vi "Main.vi"(8 "error in (no error)":errorcluster, 11 "Cascade512Base in":refnum<class "DAQCascade512.lvclass">) -> (0 "error out":errorcluster, 3 "component":refnum<class "DAQCascade512.lvclass">)   [LabVIEW 2012, in "DAQCascade512.lvclass"]
doc: "Main VI of the component."
uses:
  DAQCascade512.lvclass
  <vilib>/Distrio/Murmex/Murmex/command_enum.ctl
  <vilib>/Distrio/Murmex/InitialiseMessage/InitialiseMessage class.ctl
  <vilib>/Distrio/Murmex/InitialiseMessage/InitialiseMessage.lvclass
  DAQCascade512.lvclass/DAQCascade512.ctl
  <vilib>/Distrio/Murmex/TerminateMessage/TerminateMessage class.ctl
  <vilib>/Distrio/Murmex/TerminateMessage/TerminateMessage.lvclass
  <vilib>/Distrio/Murmex/ConfigureMessage/ConfigureMessage.lvclass
  <vilib>/Distrio/Murmex/StartMessage/StartMessage.lvclass
  <vilib>/Distrio/Murmex/StopMessage/StopMessage.lvclass
  <vilib>/Distrio/Murmex/Murmex/Set configure at initialise.vi
  <vilib>/Distrio/Murmex/Murmex/Set log reference.vi
  <vilib>/Distrio/Murmex/Murmex/Set VI reference.vi
  <vilib>/Distrio/Murmex/Murmex/Murmex.lvclass
  <vilib>/Distrio/Murmex/Message/Message.lvclass
panel:
  in  "image handles":u32[](array[numeric])
  in  "button:acquire":bool
  in  "button:stop":bool
  in  "button:start":bool
  out "img":sgl[][](graph)
  in  "button:configure":bool
  in  "Tab Control":enum32{"Settings", "Debug", "About"}(tab)
  in  "exposure":dbl=0.01 format="%.3f"
  in  "number of images":u32=1000
  out "Log":string
  out "generic command":string
  in  "command":T1
  in  "component ID":string
  in  "button:send":bool
  in  "quit":bool
  out "terminate?":bool
  # "camera made by Ali"
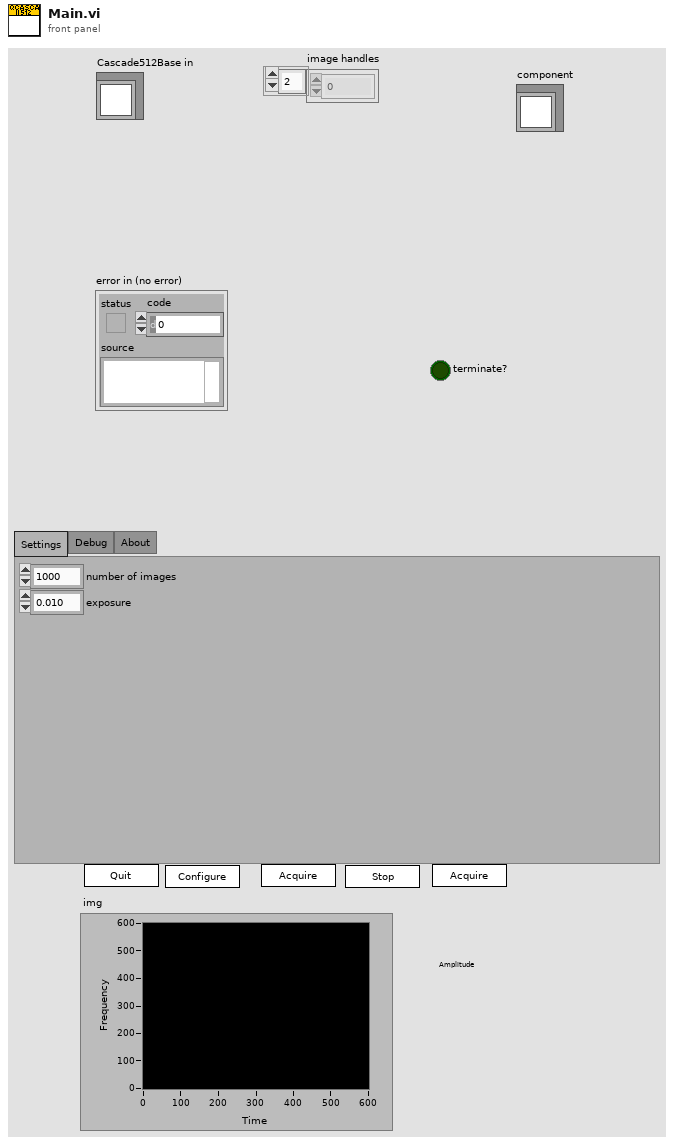
[diagram p1: front panel]
types:
  T1 = typedef "Murmex.lvlib/Murmex.lvclass/command_enum.ctl" = enum16{"null", "initialise", "reset", "terminate", "acknowledge", "update", "inspect", "inform", "proceed", "start", "stop", "fetch", "configure", "generic"}
  T2 = typedef "Murmex.lvlib/InitialiseMessage.lvclass/InitialiseMessage class.ctl" = refnum<class "InitialiseMessage.lvclass">
  T3 = typedef "Murmex.lvlib/TerminateMessage.lvclass/TerminateMessage class.ctl" = refnum<class "TerminateMessage.lvclass">
  T4 = typedef "Image_type.ctl" = u32
  T5 = typedef "Murmex.lvlib/Murmex.lvclass/Event type enumerations.ctl" = enum16{"before", "after"}
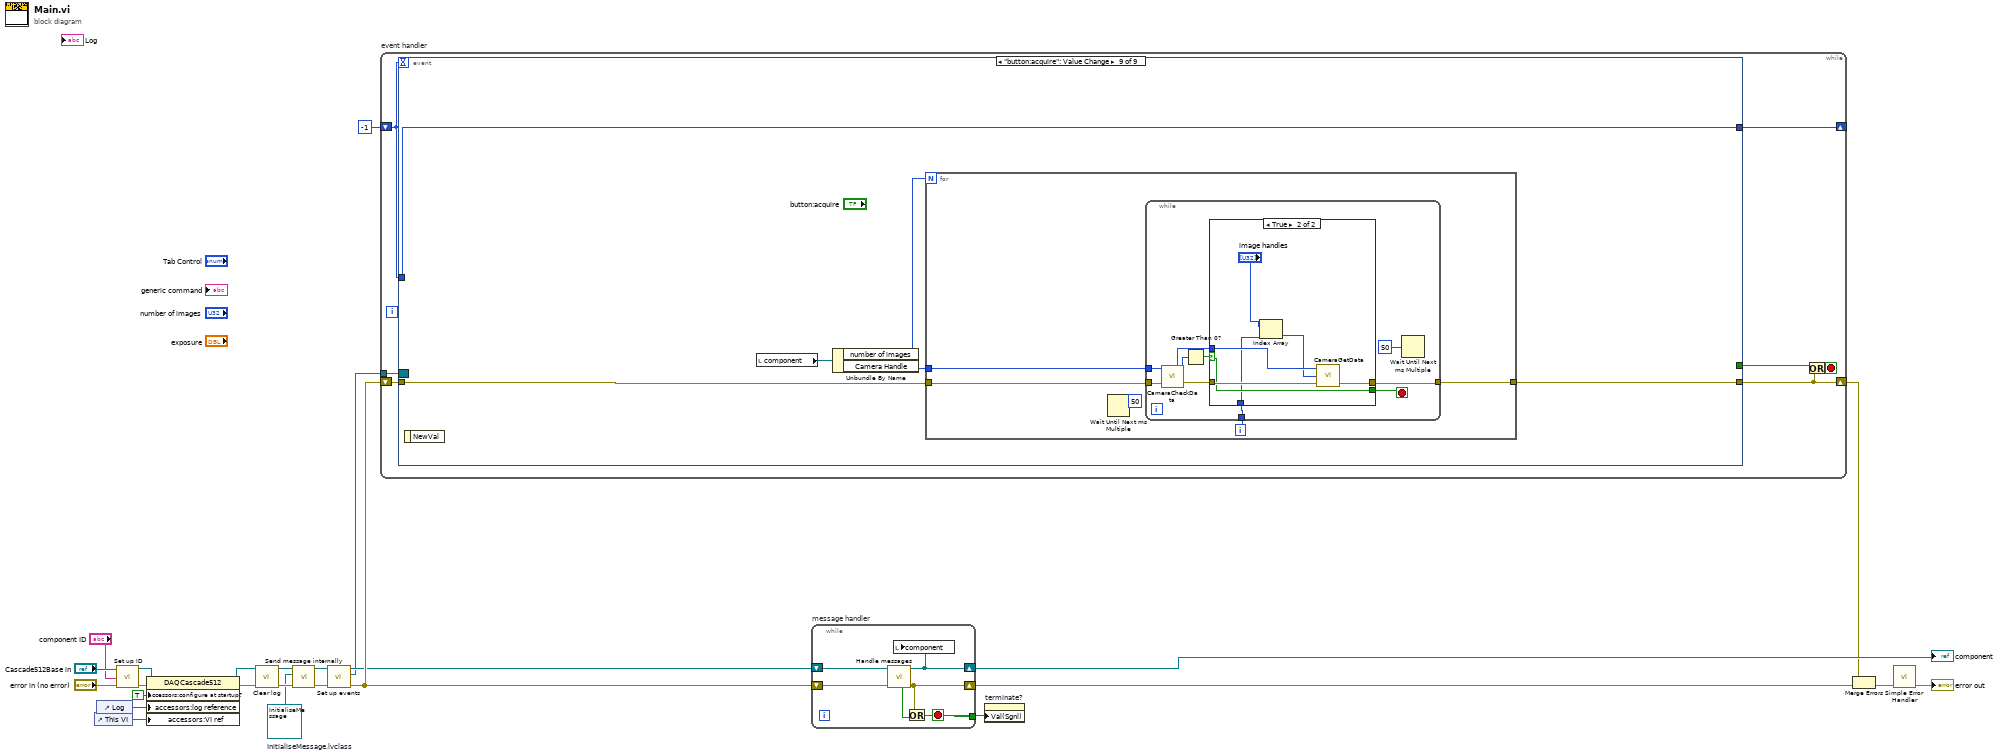
[diagram p0: block diagram]
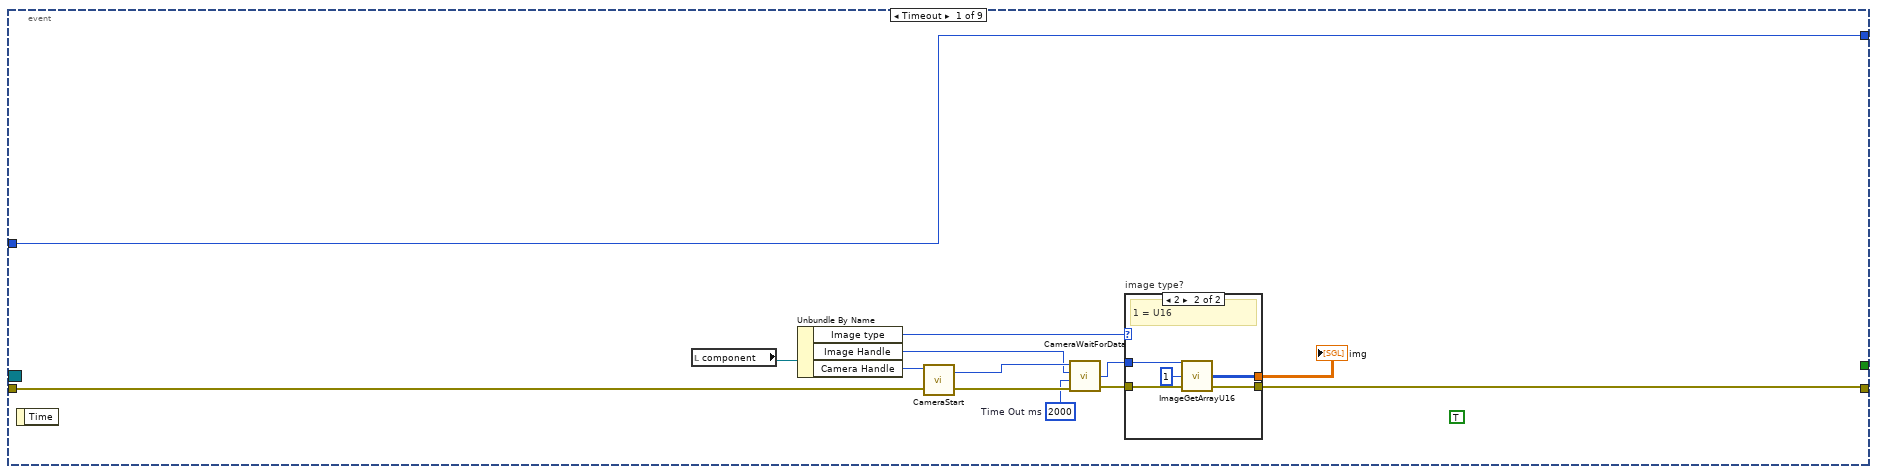
[diagram p2: hidden frame]
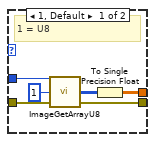
[diagram p3: hidden frame]
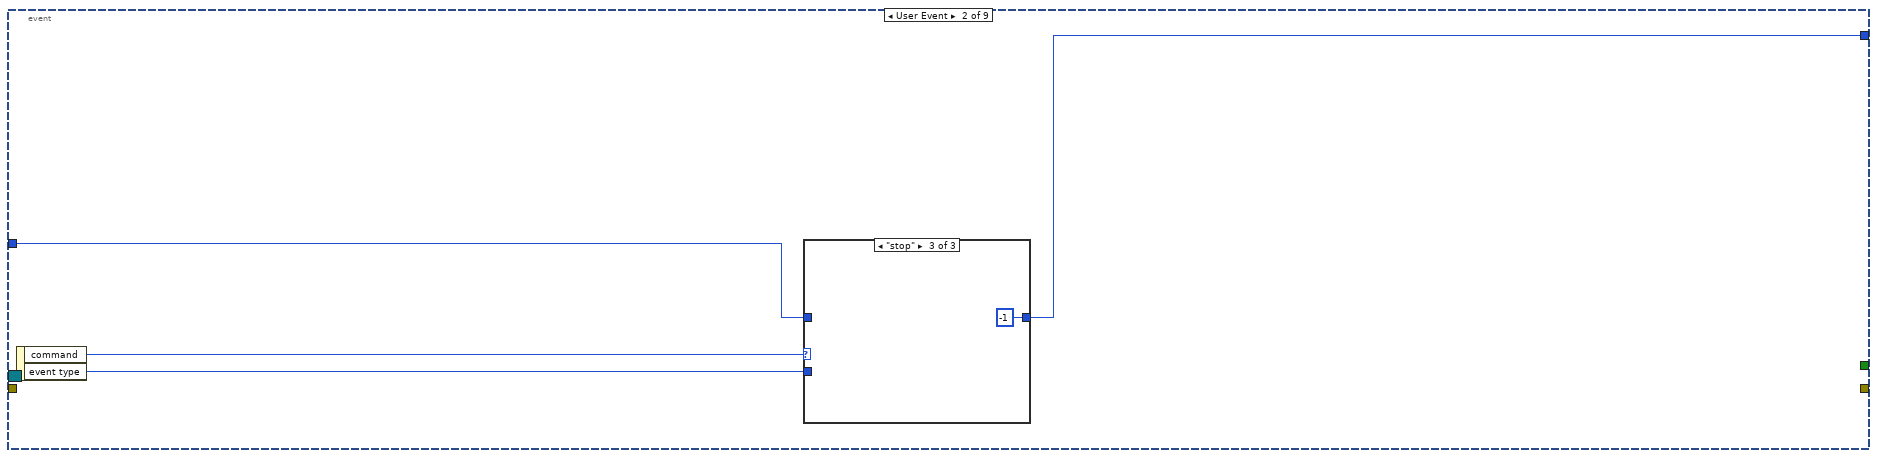
[diagram p4: hidden frame]
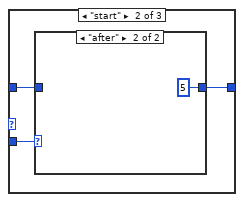
[diagram p6: hidden frame]
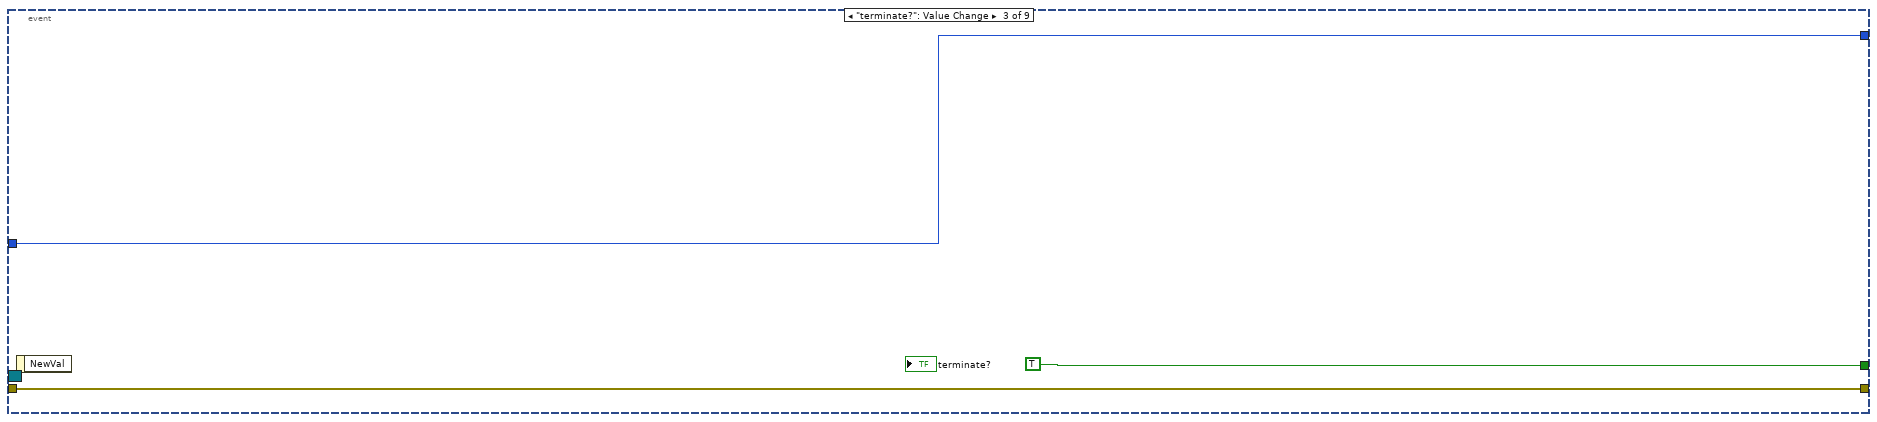
[diagram p8: hidden frame]
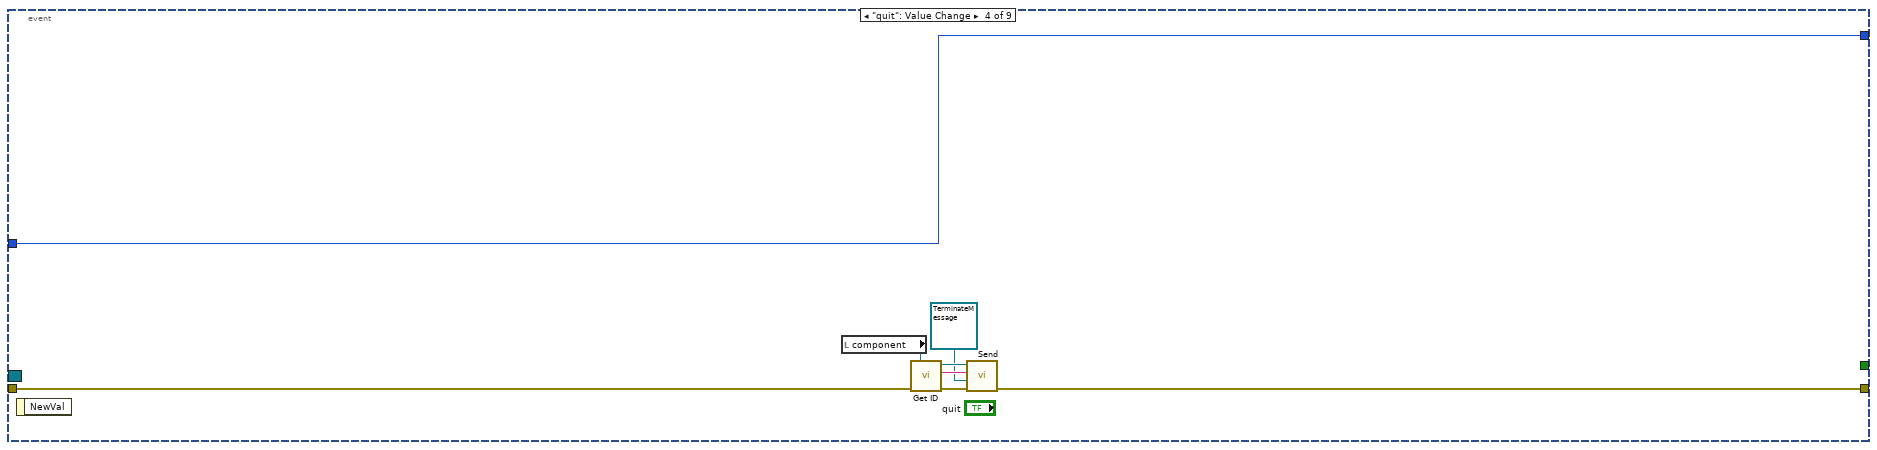
[diagram p9: hidden frame]
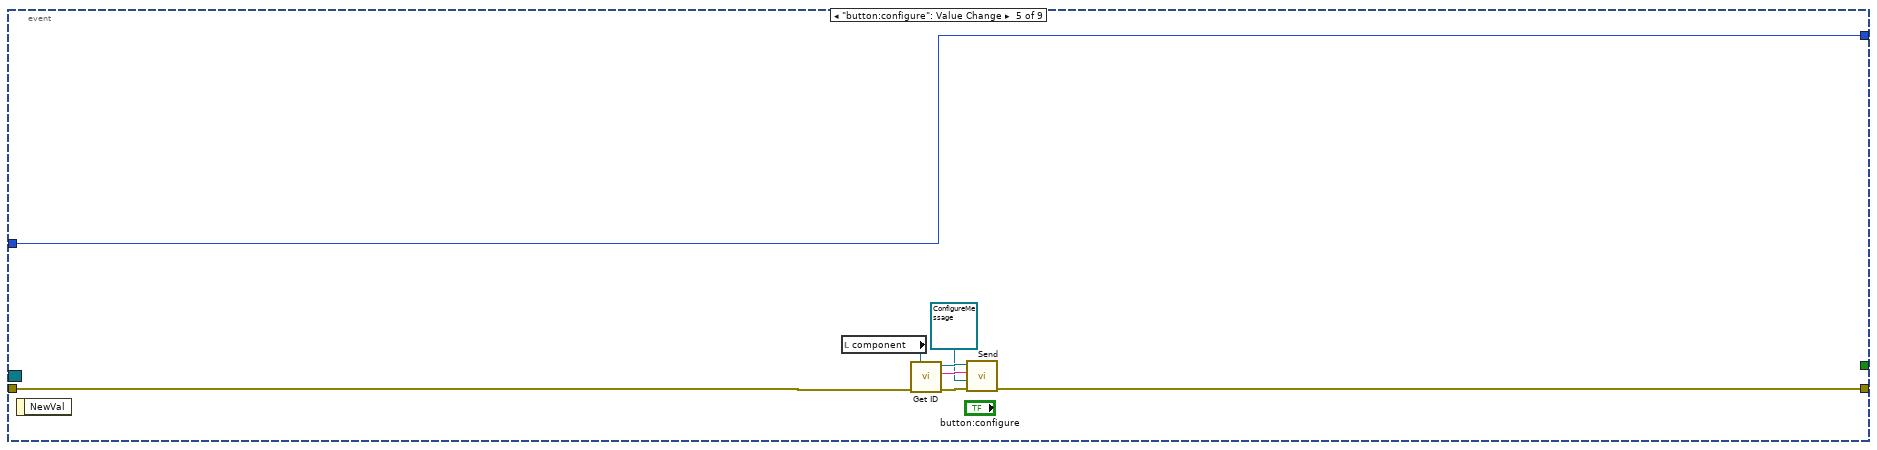
[diagram p10: hidden frame]
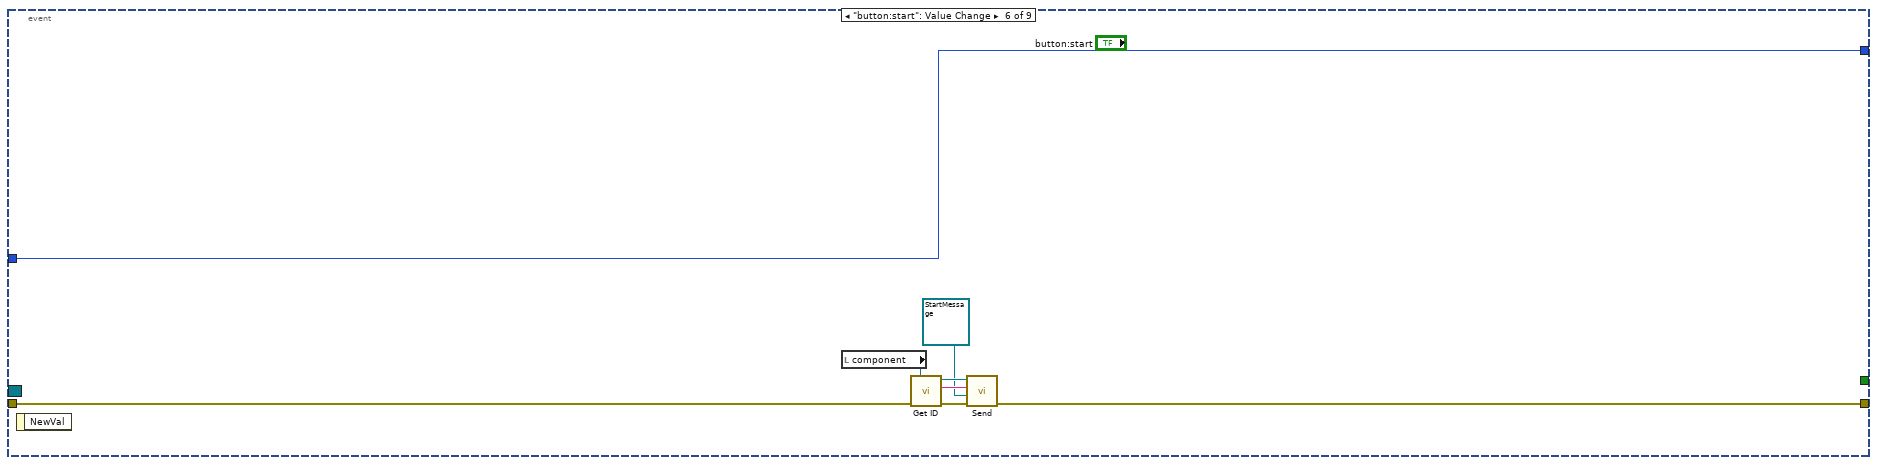
[diagram p11: hidden frame]
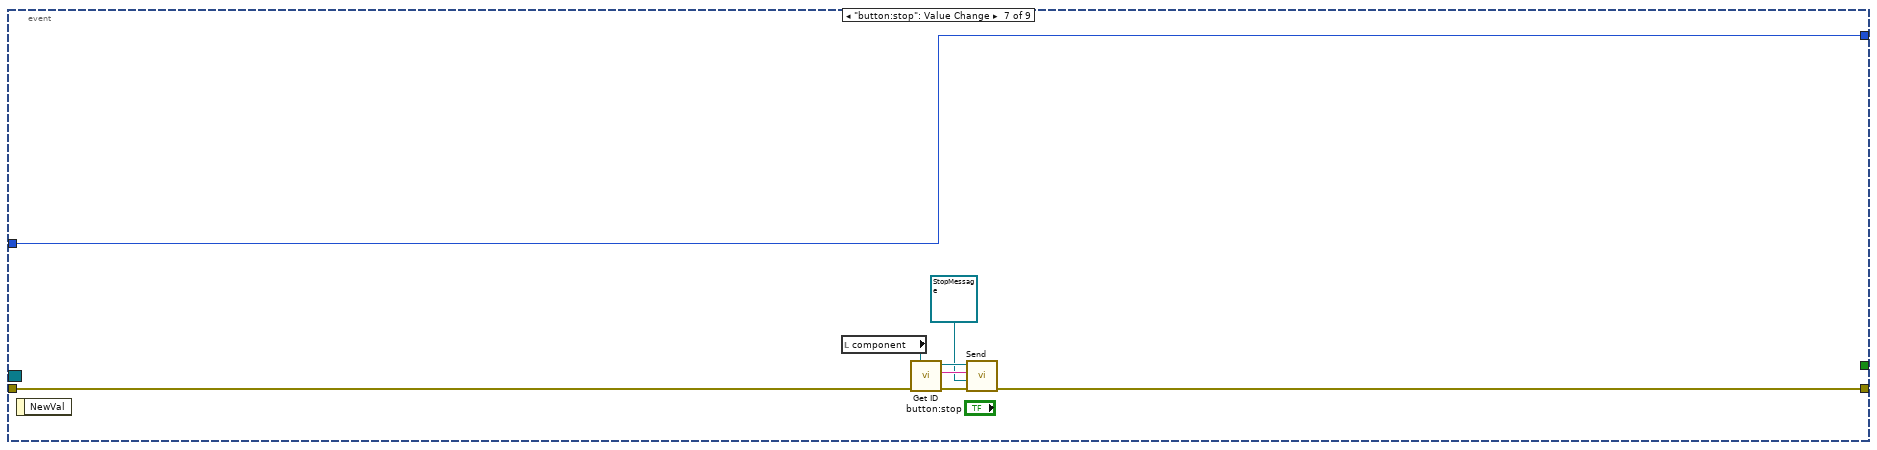
[diagram p12: hidden frame]
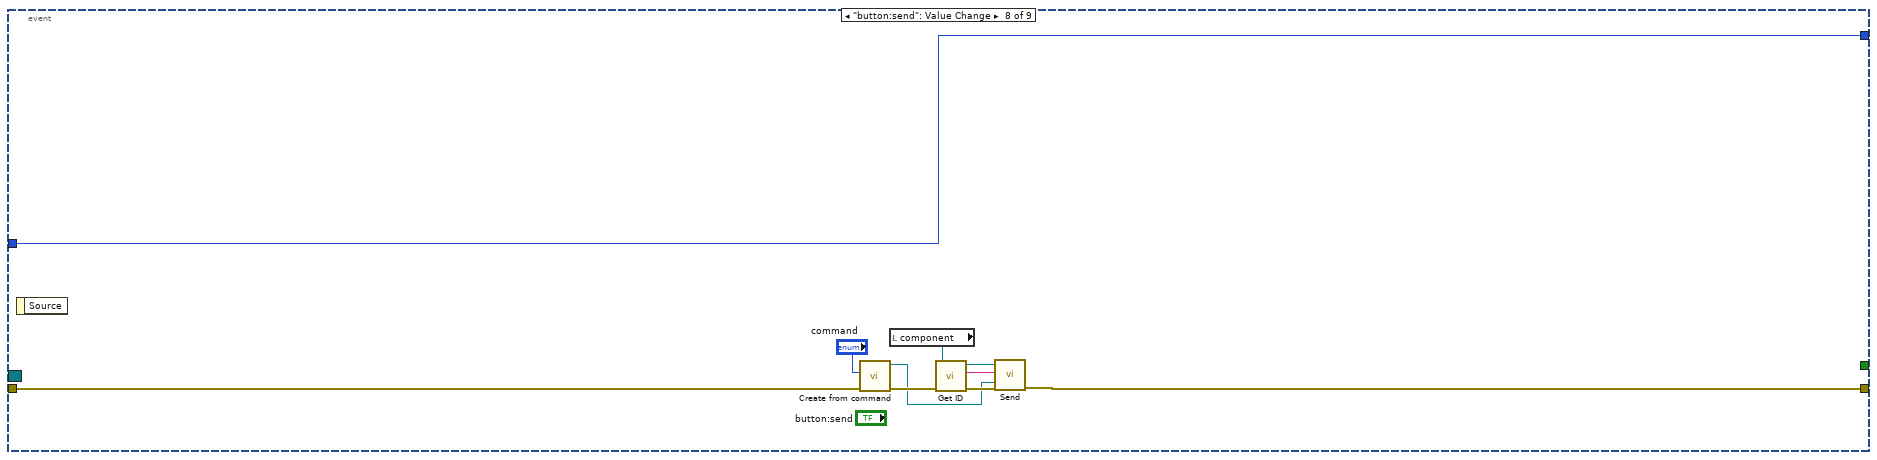
[diagram p13: hidden frame]
diagram:
  w17 = T2 refnum  # InitialiseMessage.lvclass
  n1 = control-ref of="This VI"() -> (w23:refnum<vi>)
  n2 = control-ref of="Log"() -> (w22:refnum<vi>)
  n3 = call <vilib>:"Set up ID.vi"("error in (no error)"="error in (no error)", "component ID"="component ID", "MurmexBase in"="Cascade512Base in") -> ("error out"=w13:errorcluster, "MurmexBase out"=w15:refnum<class "DAQCascade512.lvclass">)  [unwired: 6 in, 1 out]
  n4 = property class="DAQCascade512"(reference=w15, error in=w13, "accessors:configure at startup?"=TRUE, "accessors:log reference"=w22, "accessors:VI ref"=w23) -> (reference out=w21:refnum<class "DAQCascade512.lvclass">, error out=w20:errorcluster)
  n5 = call <vilib>:"Clear log.vi"("error in (no error)"=w20, "MurmexBase in"=w21) -> ("error out"=w18:errorcluster, "MurmexBase out"=w19:refnum<class "DAQCascade512.lvclass">)  [unwired: 8 in]
  n6 = call <vilib>:"Send message internally.vi"("error in (no error)"=w18, "Message"=w17, "Murmex in"=w19) -> ("error out"=w6:errorcluster, "Murmex out"=w4:refnum<class "DAQCascade512.lvclass">)  [unwired: 7 in]
  n7 = call <vilib>:"Set up events.vi"("error in (no error)"=w6, "MurmexBase in"=w4) -> ("error out"=w5:errorcluster, "Event Registration Refnum"=w2:refnum<event-registration>, "MurmexBase out"=w3:refnum<class "DAQCascade512.lvclass">)  [unwired: 7 in]
  n8 = while "event handler" {
    shift-right: [w29] -> w10
    shift-left: w5 -> [w31]
    tunnel: w2 -> [w28]
    shift-right: [w26] -> _
    shift-left: -1 -> [w27]
    stop <- w32 stop-if-true
    n9 = event shown="[8] \"button:acquire\": Value Change" {
      selector: w28 -> [_ _ _ _ _ _ _ _ _]
      dyn-events: _ -> [_ _ _ _ _ _ _ _ _]
      timeout: w27 -> [_ _ _ _ _ _ _ _ _]
      tunnel: [_ _ TRUE _ _ _ _ _ _] -> w30
      tunnel: w31 -> [w43 _ w69 w76 w84 w92 w100 w111 w117]
      tunnel: [w42 _ w69 w75 w83 w91 w99 w108 w116] -> w29
      tunnel: w27 -> [w45 w58 w68 w71 w79 w88 w96 w103 w118]
      tunnel: [w45 w57 w68 w71 w79 w88 w96 w103 w118] -> w26
      event Timeout {
        w36 = u32 2000  # Time Out ms
        (unwired) TRUE
        n10 = event-data() -> ()  [unwired: 1 in, 1 out]
        n11 = local read "component"() -> (w44:refnum<class "DAQCascade512.lvclass">)
        n12 = Unbundle By Name(w44) -> ("Image type"=w37:T4, "Image Handle"=w38:u32, "Camera Handle"=w40:u32)
        n13 = call <userlib>:"CameraStart.vi"("error in"=w43, "Camera Handle"=w40) -> ("error out"=w41:errorcluster, "Camera Handle"=w39:u32)
        n14 = call <userlib>:"CameraWaitForData.vi"("error in"=w41, "Time Out ms"=w36, "Image Handle"=w38, "Camera Handle"=w39) -> ("error out"=w35:errorcluster, "Image Handle"=w34:u32)  [unwired: 1 out]
        n15 = case "image type?" shown="2" w37 {
          tunnel: [w51 w56] -> w42
          tunnel: [w47 w55] -> w33
          tunnel: w35 -> [w49 w54]
          tunnel: w34 -> [w48 w53]
          frame 1, Default {
            # "1 = U8"
            n16 = call <userlib>:"ImageGetArrayU8.vi"("error in (no error)"=w49, "Z Position"=u32 1, "Image Handle"=w48) -> ("error out"=w51:errorcluster, "Array"=w50:u8[][])  [unwired: 1 out]
            n17 = To Single Precision Float(number=w50) -> (single precision float=w47:sgl[][])
          }
          frame 2 {
            # "1 = U16"
            n18 = call <userlib>:"ImageGetArrayU16.vi"("error in"=w54, "Z position"=u32 1, "Image Handle"=w53) -> ("error out"=w56:errorcluster, "Array uint 16"=w55:u16[][])  [unwired: 1 out]
          }
        }
        "img" <- w33
      }
      event User Event {
        n19 = event-data() -> ("command"=w60:T1, "event type"=w59:T5)  [unwired: 1 in]
        n20 = case shown="\"stop\"" w60 {
          tunnel: w59 -> [_ w64 _]
          tunnel: w58 -> [w61 w63 _]
          tunnel: [w61 w62 -1] -> w57
          frame Default {
          }
          frame "start" {
            n21 = case shown="\"after\"" w64 {
              tunnel: w63 -> [w65 _]
              tunnel: [w65 5] -> w62
              frame "before", Default {
              }
              frame "after" {
              }
            }
          }
          frame "stop" {
          }
        }
      }
      event "terminate?": Value Change {
        n22 = event-data() -> ()  [unwired: 1 in, 1 out]
      }
      event "quit": Value Change {
        n23 = event-data() -> ()  [unwired: 1 in, 1 out]
        n24 = local read "component"() -> (w74:refnum<class "DAQCascade512.lvclass">)
        n25 = call <vilib>:"Get ID.vi"("error in (no error)"=w76, "Murmex in"=w74) -> ("error out"=w78:errorcluster, "component id"=w73:string, "Murmex out"=w77:refnum<class "DAQCascade512.lvclass">)  [unwired: 7 in]
        n26 = call <vilib>:"Send.vi"("error in (no error)"=w78, "Message"=T3 refnum ("TerminateMessage.lvclass"), "recipient"=w73, "Murmex in"=w77) -> ("error out"=w75:errorcluster)  [unwired: 6 in, 1 out]
      }
      event "button:configure": Value Change {
        n27 = event-data() -> ()  [unwired: 1 in, 1 out]
        n28 = local read "component"() -> (w82:refnum<class "DAQCascade512.lvclass">)
        n29 = call <vilib>:"Get ID.vi"("error in (no error)"=w84, "Murmex in"=w82) -> ("error out"=w86:errorcluster, "component id"=w81:string, "Murmex out"=w85:refnum<class "DAQCascade512.lvclass">)  [unwired: 7 in]
        n30 = call <vilib>:"Send.vi"("error in (no error)"=w86, "Message"=refnum<class "ConfigureMessage.lvclass"> refnum ("Distrio Murmex 1.5:ConfigureMessage"), "recipient"=w81, "Murmex in"=w85) -> ("error out"=w83:errorcluster)  [unwired: 6 in, 1 out]
      }
      event "button:start": Value Change {
        n31 = event-data() -> ()  [unwired: 1 in, 1 out]
        n32 = local read "component"() -> (w90:refnum<class "DAQCascade512.lvclass">)
        n33 = call <vilib>:"Get ID.vi"("error in (no error)"=w92, "Murmex in"=w90) -> ("error out"=w94:errorcluster, "component id"=w89:string, "Murmex out"=w93:refnum<class "DAQCascade512.lvclass">)  [unwired: 7 in]
        n34 = call <vilib>:"Send.vi"("error in (no error)"=w94, "Message"=refnum<class "StartMessage.lvclass"> refnum ("Distrio Murmex 1.5:StartMessage"), "recipient"=w89, "Murmex in"=w93) -> ("error out"=w91:errorcluster)  [unwired: 6 in, 1 out]
      }
      event "button:stop": Value Change {
        n35 = event-data() -> ()  [unwired: 1 in, 1 out]
        n36 = local read "component"() -> (w98:refnum<class "DAQCascade512.lvclass">)
        n37 = call <vilib>:"Get ID.vi"("error in (no error)"=w100, "Murmex in"=w98) -> ("error out"=w102:errorcluster, "component id"=w97:string, "Murmex out"=w101:refnum<class "DAQCascade512.lvclass">)  [unwired: 7 in]
        n38 = call <vilib>:"Send.vi"("error in (no error)"=w102, "Message"=refnum<class "StopMessage.lvclass"> refnum ("Distrio Murmex 1.5:StopMessage"), "recipient"=w97, "Murmex in"=w101) -> ("error out"=w99:errorcluster)  [unwired: 6 in, 1 out]
      }
      event "button:send": Value Change {
        n39 = event-data() -> ()  [unwired: 1 in, 1 out]
        n40 = call <vilib>:"Create from command.vi"("error in (no error)"=w111, "command"="command") -> ("error out"=w110:errorcluster, "Message out"=w106:refnum<class "Message.lvclass">)  [unwired: 8 in]
        n41 = local read "component"() -> (w107:refnum<class "DAQCascade512.lvclass">)
        n42 = call <vilib>:"Get ID.vi"("error in (no error)"=w110, "Murmex in"=w107) -> ("error out"=w109:errorcluster, "component id"=w104:string, "Murmex out"=w105:refnum<class "DAQCascade512.lvclass">)  [unwired: 7 in]
        n43 = call <vilib>:"Send.vi"("error in (no error)"=w109, "Message"=w106, "recipient"=w104, "Murmex in"=w105) -> ("error out"=w108:errorcluster)  [unwired: 6 in, 1 out]
      }
      event "button:acquire": Value Change {
        n44 = event-data() -> ()  [unwired: 1 in, 1 out]
        n45 = local read "component"() -> (w115:refnum<class "DAQCascade512.lvclass">)
        n46 = Unbundle By Name(w115) -> ("number of images"=w114:u32, "Camera Handle"=w113:u32)
        n47 = for {
          N: w114 -> [_]
          tunnel: w117 -> [w123]
          tunnel: [w120] -> w116
          tunnel: w113 -> [w119]
          i -> [w121]
          n48 = Wait Until Next ms Multiple(millisecond multiple=u32 50) -> ()  [unwired: 1 out]
          n49 = while {
            tunnel: w123 -> [w132]
            tunnel: w119 -> [w131]
            tunnel: [w126] -> w120
            tunnel: w121 -> [w124]
            stop <- w127 stop-if-true
            n50 = call <userlib>:"CameraCheckData.vi"("Camera Handle"=w131, "error in"=w132) -> ("Camera Handle"=w129:u32, "Number Of Frames Available"=w133:i32, "error out"=w128:errorcluster)
            n51 = Greater Than 0?(x=w133) -> (x > 0?=w130:bool)
            n52 = case shown="True" w130 {
              selector: w130 -> [w134 w140]
              tunnel: w129 -> [_ w142]
              tunnel: w128 -> [w135 w141]
              tunnel: [w134 w140] -> w127
              tunnel: [w135 w139] -> w126
              tunnel: w124 -> [_ w138]
              frame False {
              }
              frame True {
                n53 = Index Array(array="image handles", index=w138) -> (element=w136:u32)
                n54 = call <userlib>:"CameraGetData.vi"("error in"=w141, "Data Handle"=w136, "Camera Handle"=w142) -> ("error out"=w139:errorcluster)  [unwired: 2 out]
              }
            }
            n55 = Wait Until Next ms Multiple(millisecond multiple=u32 50) -> ()  [unwired: 1 out]
          }
        }
      }
    }
    n56 = Or(x=w30, y=w29) -> (x .or. y?=w32:bool)
  }
  n57 = while "message handler" {
    shift-right: [w143] -> w25
    shift-left: w3 -> [w147]
    shift-right: [w146] -> w9
    shift-left: w5 -> [w148]
    tunnel: [w144] -> w12
    stop <- w144 stop-if-true
    n58 = call <vilib>:"Handle messages.vi"("error in (no error)"=w148, "Murmex in"=w147) -> ("error out"=w146:errorcluster, "Murmex out"=w143:refnum<class "DAQCascade512.lvclass">, "terminated?"=w145:bool)  [unwired: 7 in]
    n59 = local write "component"(w143) -> ()
    n60 = Or(x=w146, y=w145) -> (x .or. y?=w144:bool)
  }
  "component" <- w25
  n61 = property on="terminate?" class="Bool (strict)"("Val(Sgnl)"=w12) -> ()  [unwired: 2 in, 2 out]
  n62 = Merge Errors(w10, w9) -> (w8:errorcluster)
  n63 = call <vilib>:"Simple Error Handler.vi"("error in (no error)"=w8) -> ("error out"=→"error out":errorcluster)  [unwired: 4 in, 4 out]
